vi "Run.vi"(7 "Team Index":i32, 8 "Column":i32, 9 "Row":i32, 10 "View":i32[](array[numeric]) caption="View (Team Index, -1: empty)", 11 "Hail In":refnum<class "Hail.lvclass">) -> (0 "Replicated":refnum<class "Square.lvclass">, 1 "Direction":T1, 2 "Action":T2, 3 "Square Out":refnum<class "Square.lvclass">)   [LabVIEW 2015, in "Hail.lvclass"]
uses:
  Hail.lvclass
  Square/Square.lvclass
  Type Defs/Action Enum.ctl
  Type Defs/Direction Enum.ctl
  Mode Enum.ctl
  Hail.lvclass/Hail.ctl
  Group Cluster.ctl
  SubVIs/Read-Only Globals.vi
  SubVIs/Globals (private).vi
  Type Defs/SB Type Defs.lvlib
panel:
  # "NW\nN\nNE\nE\nSE\nS\nSW\nW"
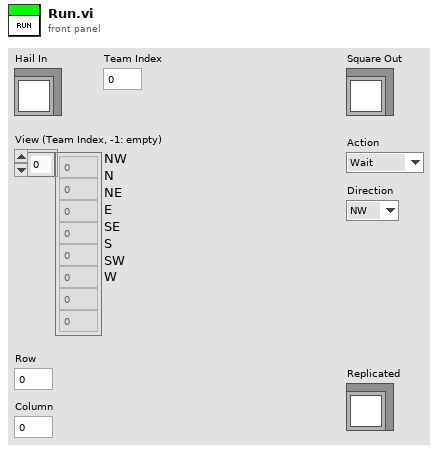
[diagram p1: front panel]
types:
  T1 = typedef "SB Type Defs.lvlib/Direction Enum.ctl" = enum16{"NW", "N", "NE", "E", "SE", "S", "SW", "W"}
  T2 = typedef "SB Type Defs.lvlib/Action Enum.ctl" = enum16{"Wait", "Move", "Attack", "Replicate"}
  T3 = typedef "Hail.lvclass/Mode Enum.ctl" = enum16{"Grow(1)", "Grow(2)", "Grow(4)", "Grow(8)", "Divide", "Farewell", "Move"}
  T4 = typedef "Hail.lvclass/Group Cluster.ctl" = cluster{"Mode":T3, "Move Amt":i32, "Group Cnt":i32, "Temp":u32, "Round":i32}
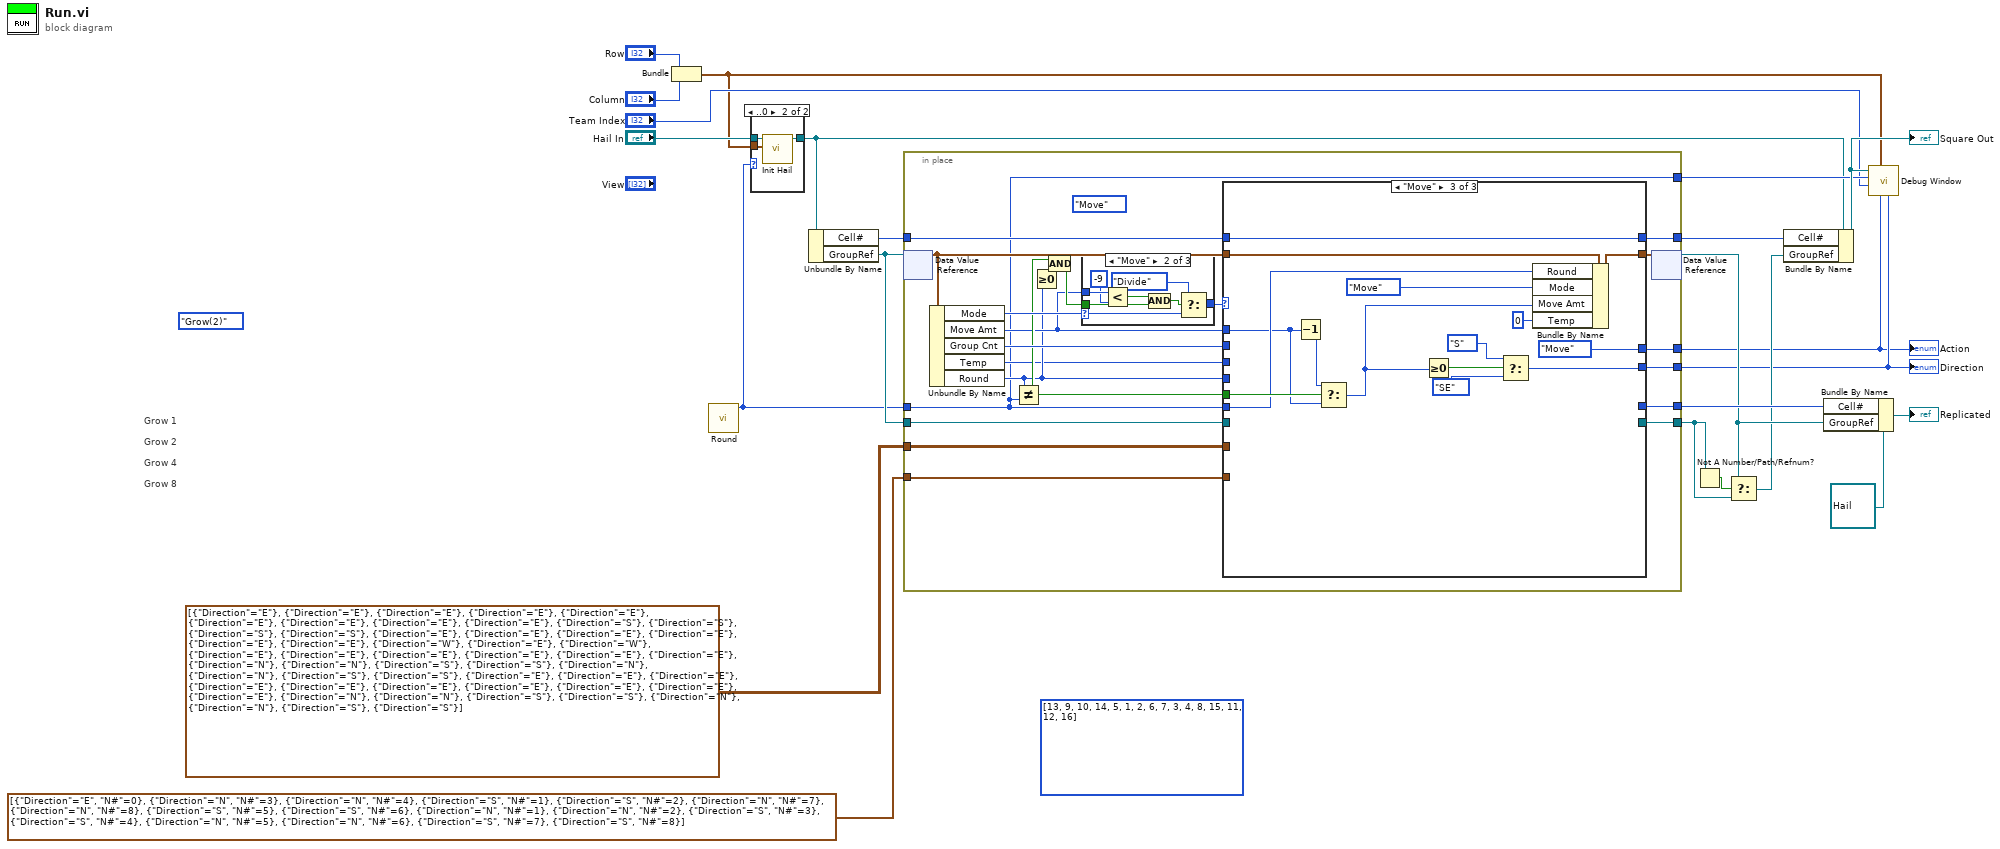
[diagram p0: block diagram]
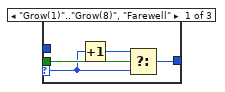
[diagram p3: hidden frame]
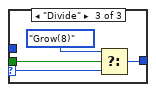
[diagram p4: hidden frame]
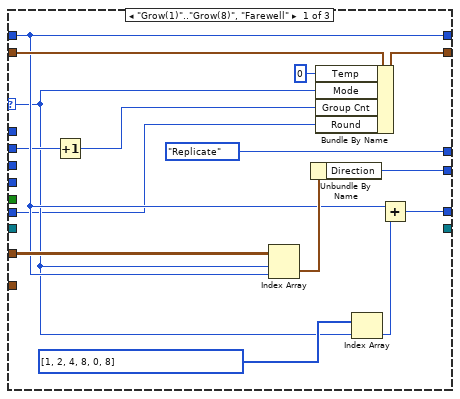
[diagram p5: hidden frame]
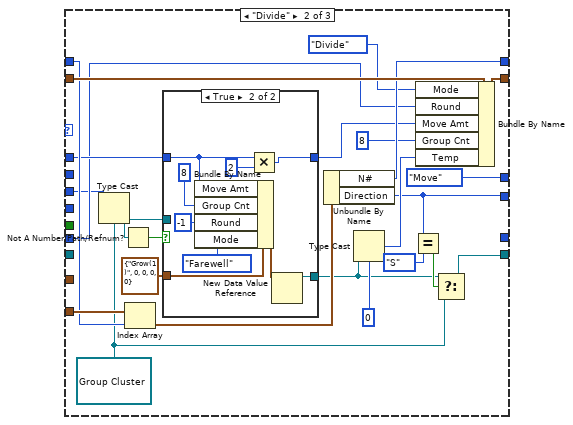
[diagram p6: hidden frame]
diagram:
  (unwired) i32[][] [[13, 9, 10, 14], [5, 1, 2, 6], [7, 3, 4, 8], [15, 11, 12, 16]]
  (unwired) Mode_Enum."Grow(2)" ("Mode")
  # "Grow 1\n\nGrow 2\n\nGrow 4\n\nGrow 8"
  n1 = Bundle("Row"="Row", "Column"="Column") -> (w3:cluster{"Row":i32, "Column":i32})  [unwired: 1 in]
  n2 = call "Round.vi"() -> ("Round"=w1:i32)  [unwired: 11 in]
  n3 = case shown="..0" w1 {
    tunnel: "Hail In" -> [w24 w27]
    tunnel: w3 -> [_ w26]
    tunnel: [w24 w25] -> w2
    frame 1.. {
    }
    frame ..0 {
      n4 = call "Init Hail.vi"("Start Player"=w26, "Hail in"=w27) -> ("Hail out"=w25:refnum<class "Hail.lvclass">)  [unwired: 8 in, 1 out]
    }
  }
  n5 = Unbundle By Name(w2) -> ("Cell#"=w23:i8, "GroupRef"=w17:refnum<data-value>)
  n6 = in-place {
    in-place-border: w23 -> [w46]
    in-place-border: [w45] -> w22
    in-place-border: [w44] -> w9
    in-place-border: [w43] -> w10
    in-place-border: cluster{"Direction":T1}[][] [[{"Direction"=enum."E"}, {"Direction"=enum."E"}, {"Direction"=enum."E"}, {"Direction"=enum."E"}, {"Direction"=enum."E"}, {"Direction"=enum."E"}, {"Direction"=enum."E"}, {"Direction"=enum."E"}, {"Direction"=enum."E"}], [{"Direction"=enum."S"}, {"Direction"=enum."S"}, {"Direction"=enum."S"}, {"Direction"=enum."S"}, {"Direction"=enum."E"}, {"Direction"=enum."E"}, {"Direction"=enum."E"}, {"Direction"=enum."E"}, {"Direction"=enum."E"}], [{"Direction"=enum."E"}, {"Direction"=enum."W"}, {"Direction"=enum."E"}, {"Direction"=enum."W"}, {"Direction"=enum."E"}, {"Direction"=enum."E"}, {"Direction"=enum."E"}, {"Direction"=enum."E"}, {"Direction"=enum."E"}], [{"Direction"=enum."E"}, {"Direction"=enum."N"}, {"Direction"=enum."N"}, {"Direction"=enum."S"}, {"Direction"=enum."S"}, {"Direction"=enum."N"}, {"Direction"=enum."N"}, {"Direction"=enum."S"}, {"Direction"=enum."S"}], [{"Direction"=enum."E"}, {"Direction"=enum."E"}, {"Direction"=enum."E"}, {"Direction"=enum."E"}, {"Direction"=enum."E"}, {"Direction"=enum."E"}, {"Direction"=enum."E"}, {"Direction"=enum."E"}, {"Direction"=enum."E"}], [{"Direction"=enum."E"}, {"Direction"=enum."N"}, {"Direction"=enum."N"}, {"Direction"=enum."S"}, {"Direction"=enum."S"}, {"Direction"=enum."N"}, {"Direction"=enum."N"}, {"Direction"=enum."S"}, {"Direction"=enum."S"}]] -> [w41]
    in-place-border: [w40] -> w18
    in-place-border: w17 -> [w39]
    in-place-border: [w38] -> w16
    in-place-border: cluster{"Direction":T1, "N#":i8}[] [{"Direction"=enum."E", "N#"=0}, {"Direction"=enum."N", "N#"=3}, {"Direction"=enum."N", "N#"=4}, {"Direction"=enum."S", "N#"=1}, {"Direction"=enum."S", "N#"=2}, {"Direction"=enum."N", "N#"=7}, {"Direction"=enum."N", "N#"=8}, {"Direction"=enum."S", "N#"=5}, {"Direction"=enum."S", "N#"=6}, {"Direction"=enum."N", "N#"=1}, {"Direction"=enum."N", "N#"=2}, {"Direction"=enum."S", "N#"=3}, {"Direction"=enum."S", "N#"=4}, {"Direction"=enum."N", "N#"=5}, {"Direction"=enum."N", "N#"=6}, {"Direction"=enum."S", "N#"=7}, {"Direction"=enum."S", "N#"=8}] -> [w37]
    in-place-border: [w28] -> w8
    in-place-border: w1 -> [w28]
    (unwired) Mode_Enum."Move" ("Mode")
    n7 = in-place-dvr #1(w17) -> (w47:T4)  [unwired: 1 out]
    n8 = Unbundle By Name(w47) -> ("Mode"=w36:T3, "Move Amt"=w31:i32, "Group Cnt"=w48:i32, "Temp"=w29:u32, "Round"=w30:i32)
    n9 = Not Equal?(x=w30, y=w28) -> (x != y?=w34:bool)
    n10 = Greater Or Equal To 0?(x=w30) -> (x >= 0?=w33:bool)
    n11 = Compound Arithmetic op=AND(w34, w33) -> (w32:bool)
    n12 = case shown="\"Move\"" w36 {
      selector: w36 -> [w51 w60 w61]
      tunnel: [w49 w59 w62] -> w35
      tunnel: w32 -> [w52 w58 w64]
      tunnel: w31 -> [_ w54 _]
      frame "Grow(1)".."Grow(8)", "Farewell" {
        n13 = Increment(x=w51) -> (x+1=w50:T3)
        n14 = Select(t=w50, s=w52, f=w51) -> (s? t:f=w49:T3)
      }
      frame "Move" {
        n15 = Less?(x=w54, y=-9) -> (x < y?=w55:bool)
        n16 = Compound Arithmetic op=AND(w55, w58) -> (w57:bool)
        n17 = Select(t=Mode_Enum."Divide" ("Mode"), s=w57, f=w60) -> (s? t:f=w59:T3)
      }
      frame "Divide" {
        n18 = Select(t=Mode_Enum."Grow(8)" ("Mode"), s=w64, f=w61) -> (s? t:f=w62:T3)
      }
    }
    n19 = case shown="\"Move\"" w35 {
      selector: w35 -> [w67 _ _]
      tunnel: w31 -> [_ w95 w118]
      tunnel: w48 -> [w70 _ _]
      tunnel: w47 -> [w78 w103 w129]
      tunnel: w46 -> [w73 w99 w127]
      tunnel: [w73 w97 w127] -> w45
      tunnel: [Action_Enum."Replicate" ("Action") Action_Enum."Move" ("Action") Action_Enum."Move" ("Action")] -> w44
      tunnel: [w74 w88 w121] -> w43
      tunnel: [w77 w102 w128] -> w42
      tunnel: w41 -> [w76 _ _]
      tunnel: [w71 _ _] -> w40
      tunnel: w39 -> [_ _ _]
      tunnel: [_ w84 _] -> w38
      tunnel: w37 -> [_ w100 _]
      tunnel: w30 -> [_ _ _]
      tunnel: w28 -> [w66 w82 w119]
      tunnel: w34 -> [_ _ w120]
      tunnel: w29 -> [_ w80 _]
      frame "Grow(1)".."Grow(8)", "Farewell" {
        n20 = Increment(x=w70) -> (x+1=w69:i32)
        n21 = Index Array(array=w76, index (row)=w67, index (col)=w73) -> (element=w75:cluster{"Direction":T1})
        n22 = Unbundle By Name(w75) -> ("Direction"=w74:T1)
        n23 = Bundle By Name(cluster=w78, "Temp"=u32 0, "Mode"=w67, "Group Cnt"=w69, "Round"=w66) -> (w77:T4)
        n24 = Index Array(array=i32[] [1, 2, 4, 8, 0, 8], index=w67) -> (element=w72:i32)
        n25 = Add(x=w73, y=w72) -> (x+y=w71:i32)
      }
      frame "Divide" {
        w83 = refnum<data-value> refnum ("data value reference")
        n26 = Type Cast(type=w83, x=w80) -> (*(type *) &x=w89:refnum<data-value>)
        n27 = Not A Number/Path/Refnum?(number/path/refnum=w89) -> (NaN/Path/Refnum?=w90:bool)
        n28 = Index Array(array=w100, index=w99) -> (element=w98:cluster{"Direction":T1, "N#":i8})
        n29 = case shown="True" w90 {
          tunnel: T4 {"Mode"=enum."Grow(1)", "Move Amt"=0, "Group Cnt"=0, "Temp"=0, "Round"=0} ("Group Cluster") -> [_ w114]
          tunnel: w95 -> [w105 w106]
          tunnel: [w105 w112] -> w94
          tunnel: [w104 w108] -> w85
          tunnel: w89 -> [w104 _]
          frame False {
          }
          frame True {
            n30 = Bundle By Name(cluster=w114, "Move Amt"=w106, "Group Cnt"=8 ("y"), "Round"=-1, "Mode"=Mode_Enum."Farewell") -> (w110:T4)
            n31 = Multiply(x=w106, y=2) -> (x*y=w112:i32)
            n32 = New Data Value Reference(data value=w110) -> (data value reference=w108:refnum<data-value>)  [unwired: 1 in, 1 out]
          }
        }
        n33 = Unbundle By Name(w98) -> ("N#"=w97:i8, "Direction"=w88:T1)
        n34 = Type Cast(type=u32 0 ("Group Cnt"), x=w85) -> (*(type *) &x=w91:u32)
        n35 = Equal?(x=w88, y=Direction_Enum."S") -> (x = y?=w86:bool)
        n36 = Bundle By Name(cluster=w103, "Mode"=Mode_Enum."Divide", "Round"=w82, "Move Amt"=w94, "Group Cnt"=8, "Temp"=w91) -> (w102:T4)
        n37 = Select(t=w85, s=w86, f=w83) -> (s? t:f=w84:refnum<data-value>)
      }
      frame "Move" {
        n38 = Decrement(x=w118) -> (x-1=w126:i32)
        n39 = Select(t=w126, s=w120, f=w118) -> (s? t:f=w116:i32)
        n40 = Greater Or Equal To 0?(x=w116) -> (x >= 0?=w124:bool)
        n41 = Select(t=Direction_Enum."S" ("Direction"), s=w124, f=Direction_Enum."SE" ("Direction")) -> (s? t:f=w121:T1)
        n42 = Bundle By Name(cluster=w129, "Round"=w119, "Mode"=Mode_Enum."Move", "Move Amt"=w116, "Temp"=u32 0) -> (w128:T4)
      }
    }
    n43 = in-place-dvr #1(w42) -> (w13:refnum<data-value>)  [unwired: 1 out]
  }
  "Action" <- w9
  "Direction" <- w10
  n44 = Not A Number/Path/Refnum?(number/path/refnum=w16) -> (NaN/Path/Refnum?=w15:bool)
  n45 = Select(t=w13, s=w15, f=w16) -> (s? t:f=w12:refnum<data-value>)
  n46 = Bundle By Name(cluster=w2, "Cell#"=w22, "GroupRef"=w12) -> (w11:refnum<class "Hail.lvclass">)
  "Square Out" <- w11
  n47 = Bundle By Name(cluster=refnum<class "Hail.lvclass"> refnum ("Hail.lvclass"), "Cell#"=w18, "GroupRef"=w13) -> (→"Replicated":refnum<class "Hail.lvclass">)
  n48 = call "Debug Window.vi"("Direction"=w10, "Action"=w9, "Pos"=w3, "Team Idx"="Team Index", "Round"=w8, "Hail"=w11) -> ()  [unwired: 6 in]
